vi "Write DVR.vi"(8 "error in (no error)":errorcluster, 10 "DVR":refnum<data-value>, 11 "Crosswinds in":refnum<class "Crosswinds.lvclass">) -> (0 "error out":errorcluster, 3 "Crosswinds out":refnum<class "Crosswinds.lvclass">)   [LabVIEW 2015, in "Crosswinds.lvclass"]
uses:
  Crosswinds.lvclass
  DVR Cluster.ctl
  Spot Cluster.ctl
  State Enum.ctl
  Role Enum.ctl
  Type Defs/Direction Enum.ctl
  Crosswinds.lvclass/Crosswinds.ctl
  Type Defs/SB Type Defs.lvlib
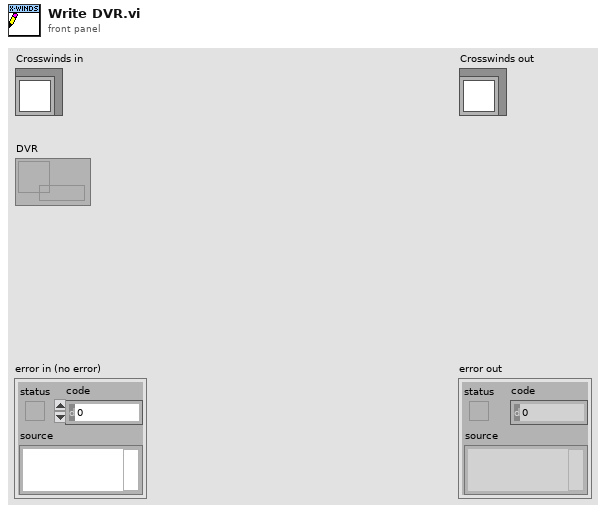
[diagram p1: front panel]
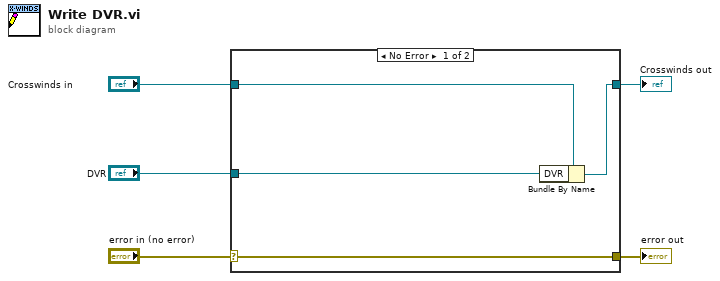
[diagram p0: block diagram]
diagram:
  n1 = case shown="No Error" "error in (no error)" {
    selector: "error in (no error)" -> [w9 w10]
    tunnel: [w9 w10] -> w4
    tunnel: [w7 w11] -> w2
    tunnel: "Crosswinds in" -> [w8 w11]
    tunnel: "DVR" -> [w6 _]
    frame No Error {
      n2 = Bundle By Name(cluster=w8, "DVR"=w6) -> (w7:refnum<class "Crosswinds.lvclass">)
    }
    frame Error {
    }
  }
  "error out" <- w4
  "Crosswinds out" <- w2
